vi "Set Hood Position.vi"(10 "Increment":bool, 11 "Decrement":bool) -> ()   [LabVIEW 2011]
uses:
  System Set Points and States.vi
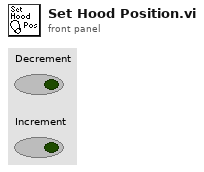
[diagram p1: front panel]
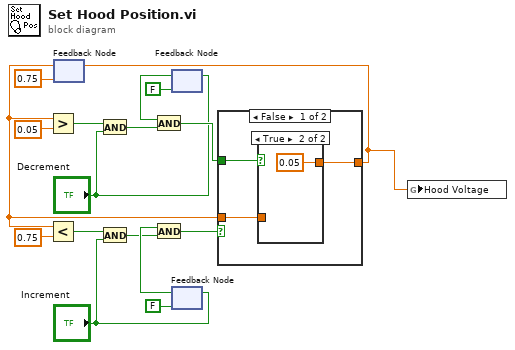
[diagram p0: block diagram]
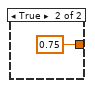
[diagram p3: hidden frame]
diagram:
  n1 = feedback #1(0.75) -> (w17:dbl)
  n2 = Greater?(x=w17, y=0.05) -> (0:w13:bool)
  n3 = Less?(x=w17, y=0.75) -> (x < y?=w4:bool)
  n4 = And(x=w13, y="Decrement") -> (x .and. y?=w12:bool)
  n5 = And(x=w4, y="Increment") -> (x .and. y?=w5:bool)
  n6 = feedback #2(FALSE ("Increment")) -> (w11:bool)
  n7 = And(x=w11, y=w12) -> (x .and. y?=w16:bool)
  n8 = feedback-in #2("Decrement") -> ()
  n9 = feedback #3(FALSE ("Increment")) -> (w8:bool)
  n10 = And(x=w8, y=w5) -> (x .and. y?=w6:bool)
  n11 = feedback-in #3("Increment") -> ()
  n12 = case shown="False" w6 {
    tunnel: w16 -> [w20 _]
    tunnel: w17 -> [w19 _]
    tunnel: [w18 0.75] -> w1
    frame False {
      n13 = case shown="True" w20 {
        tunnel: w19 -> [w21 _]
        tunnel: [w21 0.05] -> w18
        frame False {
        }
        frame True {
        }
      }
    }
    frame True {
    }
  }
  n14 = feedback-in #1(w1) -> ()
  n15 = global write "System Set Points and States.vi" "Hood Voltage"(w1) -> ()
